vi "setControllerUsbReference.vi"(8 "error in (no error)":errorcluster, 10 "reference":i32, 11 "reference (in)":refnum<class "_Controller.lvclass">) -> (0 "error out":errorcluster, 3 "reference (out)":refnum<class "_Controller.lvclass">)   [LabVIEW 2013, in "classes.lvlib" / "_Controller.lvclass"]
doc: "Produced By:\n\n<B>Kod Integrations, LLC</B>\n4835 Marianne Drive\nMount Airy, MD 21771\nhttp://www.kodintegrations.com\nemail: info@kodintegrations.com\nphone: (240) 687-1288"
uses:
  _Controller.lvclass
  _Controller.lvclass/_Controller.ctl
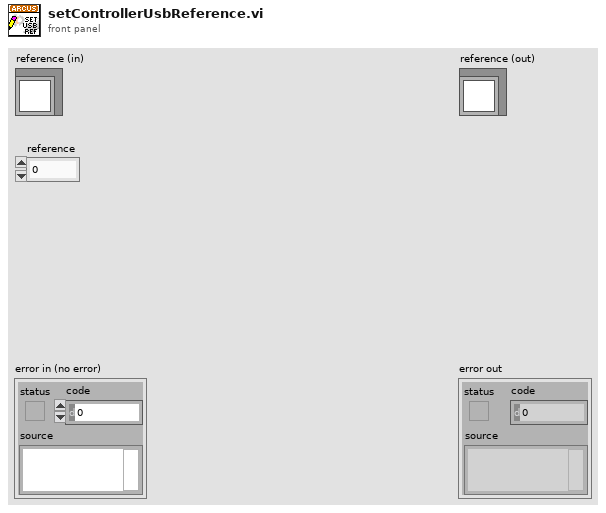
[diagram p1: front panel]
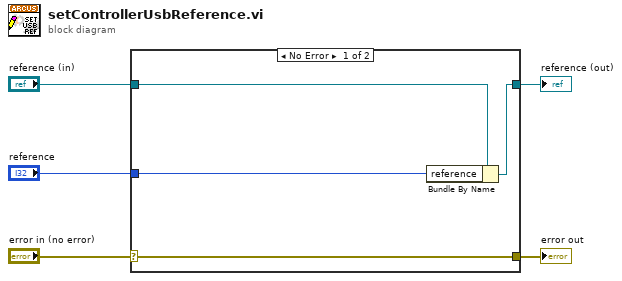
[diagram p0: block diagram]
diagram:
  n1 = case shown="No Error" "error in (no error)" {
    selector: "error in (no error)" -> [w9 w10]
    tunnel: [w9 w10] -> w4
    tunnel: [w7 w11] -> w2
    tunnel: "reference (in)" -> [w8 w11]
    tunnel: "reference" -> [w6 _]
    frame No Error {
      n2 = Bundle By Name(cluster=w8, "reference"=w6) -> (w7:refnum<class "_Controller.lvclass">)
    }
    frame Error {
    }
  }
  "error out" <- w4
  "reference (out)" <- w2
